vi "To Generic.vi"(8 "error in (no error)":errorcluster, 11 "Cluster in":refnum<class "Cluster.lvclass">) -> (0 "error out":errorcluster, 2 "Generic Data":refnum<class "Generic Data.lvclass">[](array[class]), 3 "Data Name":string[](array[string]))   [LabVIEW 2020, in "Data.lvlib" / "Cluster.lvclass"]
doc: "Present private data as an array of named generic data elements."
uses:
  Cluster.lvclass
  Generic Data.lvclass
  Cluster.lvclass/Cluster.ctl
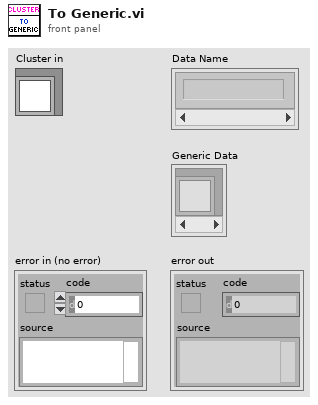
[diagram p1: front panel]
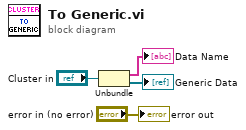
[diagram p0: block diagram]
diagram:
  n1 = Unbundle("Cluster in") -> (→"Data Name":string[], →"Generic Data":refnum<class "Generic Data.lvclass">[])
  "error out" <- "error in (no error)"
